vi "Dashboard Main.vi"() -> ()   [LabVIEW 2012]
uses:
  <vilib>/Rock Robotics/WPI/Camera/WPI_CameraWhite Balance Values.ctl
  <vilib>/event_ctls.llb/eventvkey.ctl
  <vilib>/Utility/config.llb/Read Key (String).vi
  <vilib>/Utility/config.llb/Read Key (I32).vi
  <vilib>/Utility/config.llb/Write Key (String).vi
  <vilib>/Utility/config.llb/Write Key (I32).vi
  <vilib>/Utility/inputDevices.llb/keyboardAcquire.vi
  Keys Pressed Global.vi
  <vilib>/Utility/inputDevices.llb/joystickAcquire.vi
  <vilib>/Utility/config.llb/NI_LVConfig.lvlib
panel:
  in  "Range":cluster{"Lower value":sgl, "Upper value":sgl}={"Lower value"=150.0, "Upper value"=255.0} {"Lower value" scale=0.0..255.0; "Upper value" scale=0.0..255.0}
  in  "Color Plane":i32(ring)=7 items=["Red", "Green", "Blue", "Hue", "Saturation", "Luminance", "Value", "Intensity"]
  out "Battery Value":dbl(slide) scale=0.0..14.0 scale format="%#_2e"
  out "Battery":sgl(graph)
  in  "Camera Settings":T1={"Frate Rate"=30, "Compression"=30, "Size"=0} {"Frate Rate" scale=1.0..30.0; "Size" items=["640x480", "320x240", "160x120"]}
  out "Mode":T2(ring)=enum."Auto Disabled"
  out "Camera IP":string
  out "JS1 Z":dbl(slide) scale=-1.0..1.0 scale format="%#_2e"
  out "JS2 Z":dbl(slide) scale=-1.0..1.0 scale format="%#_2e"
  out "Joystick 1":cluster{"X":dbl, "Y":dbl}[](graph)
  out "Joystick 2":cluster{"X":dbl, "Y":dbl}[](graph)
  out "JS Buttons 1":T3
  out "JS Buttons 2":T3
  out "MotorSlide4":dbl(slide) scale=-1.0..1.0 scale format="%#_2e"
  out "MotorSlide3":dbl(slide) scale=-1.0..1.0 scale format="%#_2e"
  out "MotorSlide2":dbl(slide) scale=-1.0..1.0 scale format="%#_2e"
  in  "MotorName3":string="Front Left"
  in  "MotorName4":string="Front Right"
  in  "MotorName1":string="Rear Left"
  in  "MotorName2":string="Rear Right"
  out "MotorChart4":dbl(graph)
  out "MotorChart3":dbl(graph)
  out "MotorChart2":dbl(graph)
  out "MotorSlide1":dbl(slide) scale=-1.0..1.0 scale format="%#_2e"
  out "MotorChart1":dbl(graph)
  out "Robot IP":string
  in  "Dashboard Tab":T4(tab)
  in  "control feeder":bool
  in  "control flipper":bool
  in  "conveyer backward":bool
  in  "conveyer forward":bool
  in  "transfer backward":bool
  in  "transfer forward":bool
  in  "feeder":dbl(knob) scale=0.0..130.0
  in  "flipper":dbl(knob) scale=0.0..170.0
  in  "Checkbox 2":bool
  in  "Checkbox 1":bool
  in  "Slider 1":dbl(slide) scale=0.0..100.0
  out "keys pressed":T5(array[ring])
  out "Position of Target's Center (x, y)":dbl[](array[numeric])
  out "Distance to Targets Center [m]":dbl
  out "Processed Image":T6(plugin-control)
  out "Target Found":bool
  in  "Annotate":bool=TRUE
  in  "Slider":dbl(slide) scale=0.0..100.0 scale format="%#_3g"
  in  "On/Off":bool caption="Solenoid"
  in  "Test Name":u16(ring) items=["Select the test to run...", "Example Test", "-------------------------------", "List of tests is built in robot code.", "Replace with your own automated tests."]
  in  "Test Tree":string(tree)
  in  "Motor":cluster{"Value":dbl, "Enable":bool} {"Value" scale=-1.0..1.0 scale format="%#_3g"}
  out "Progress":T7 {"Test Progress" scale=0.0..100.0}
  in  "Rev/Fwd":cluster{"Forward":bool, "Reverse":bool}
  in  "Ring":u16(ring) items=["Auto", "Fixed indoor", "Fixed outdoor 1", "Fixed outdoor 2", "Fixed fluorescent 1", "Fixed fluorescent 2", "Hold current"]
  in  "Listbox":i32(listbox)
  out "Selected Target Info":T8
  in  "Target Choice":i8(knob) scale=0.0..2.0
  in  "Viewer":enum32{"Camera Image", "Map", "Variables"}(tab)
  in  "More Cam":bool
  out "Mbps":dbl format="%#.1g"
  in  "Enable":bool
  in  "DB Camera Config":bool
  out "Mbps":bool
  out "fps":dbl format="%#.1g"
  out "Image Error Message":string="Timeout in Camera Communications"
  out "Camera Image":T6(plugin-control)
  in  "1":bool
  in  "2":bool
  in  "3":bool
  in  "Pyramid":bool
  in  "Low":bool
  in  "Left":bool
  in  "Right":bool
  in  "High":bool
  out "Map":T6(plugin-control)
  out "Distance [Meter]":dbl
  out "Angle [Degrees]":dbl
  out "Latched Cordinates":i32[](array[numeric])
  out "Selected Goal":i32
  out "Selected Cordinates":i32[](array[numeric])
  out "Tree":string(tree)
  # "Drive & Motors"
  # "Robot IP:"
  # "feeder"
  # "transfer"
  # "flipper"
  # "conveyer belt"
  # "Customize by placing controls and indicators here and name to match\nDashboard Variables on robot."
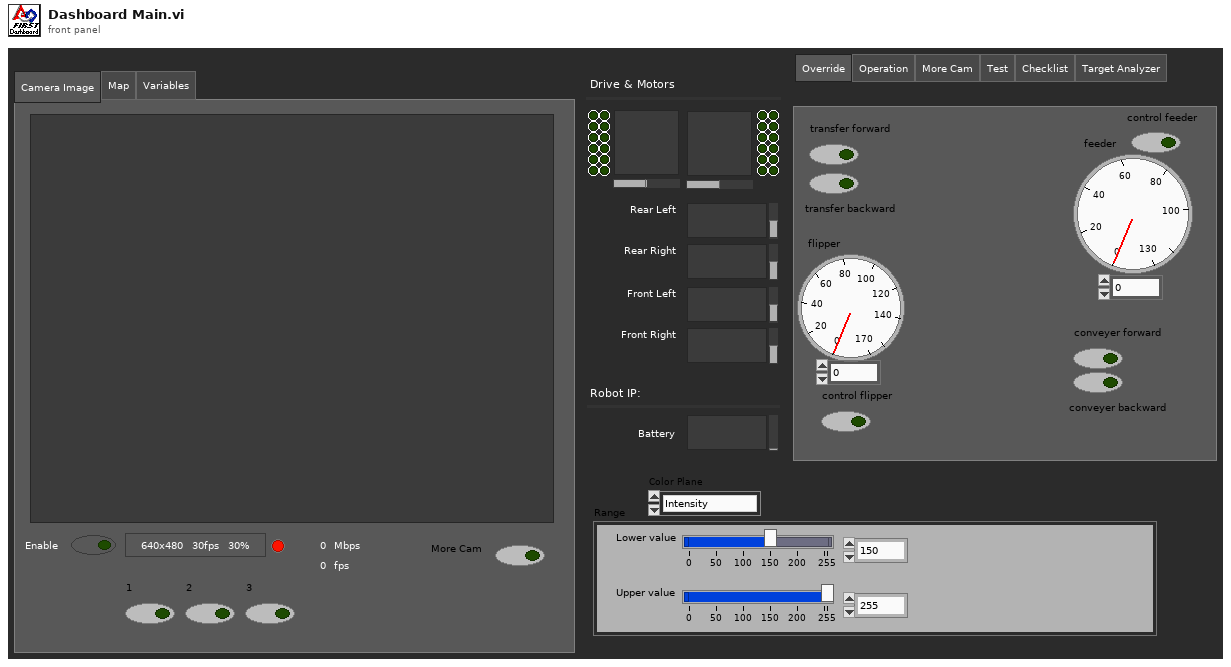
[diagram p1: front panel]
types:
  T1 = cluster{"Frate Rate":i32, "Compression":i32, "Size":u16}
  T2 = enum8{"Tele-Op Disabled", "Tele-Op Enabled", "Auto Disabled", "Auto Enabled", "Test Disabled", "Test Enabled", ""}
  T3 = cluster{bool, bool, bool, bool, bool, bool, bool, bool, bool, bool, bool, bool}
  T4 = enum32{"Override", "Operation", "More Cam", "Test", "Checklist", "Target Analyzer"}
  T5 = enum16{"0", "1", "2", "3", "4", "5", "6", "7", "8", "9", "A", "B", "C", "D", "E", "F", "G", "H", "I", "J", "K", "L", "M", "N", "O", "P", "Q", "R", "S", "T", "U", "V", "W", "X", "Y", "Z", "F1", "F2", "F3", "F4", "F5", "F6", "F7", "F8", "F9", "F10", "F11", "F12", "F13", "F14", "F15", "ADD", "BACK", "BACKSLASH", "CAPITAL", "COMMA", "DECIMAL", "DELETE", "DIVIDE", "DOWN", "END", "EQUALS", "ESCAPE", "GRAVE (`)", "HOME", "INSERT", "LBRACKET", "LCONTROL", "LEFT", "L ALT", "LSHIFT", "LWIN", "MINUS", "MULTIPLY", "NEXT", "NUMLOCK", "NUMPAD_0", "NUMPAD_1", "NUMPAD_2", "NUMPAD_3", "NUMPAD_4", "NUMPAD_5", "NUMPAD_6", "NUMPAD_7", "NUMPAD_8", "NUMPAD_9", "PAUSE", "PERIOD", "PRIOR (PG UP)", "RBRACKET", "RCONTROL", "RETURN", "RIGHT", "R ALT", "RSHIFT", "RWIN", "SCROLL", "SEMICOLON", "SLASH", "SPACE", "SUBTRACT", "TAB", "UP", "ENTER (num pad)", "' (quote)"}[]
  T6 = typedef "IMAQ Image.ctl" = refnum<image>
  T7 = cluster{"Test Progress":u8, "Test Progress Text":string}
  T8 = cluster{"Position":cluster{"X":dbl, "Y":dbl}, "Distance (m)":dbl, "Target Found?":bool}
  T9 = typedef "Image Type" = u32
  T10 = typedef "WPI_CameraWhite Balance Values.ctl" = enum16{"Auto", "Fixed indoor", "Fixed outdoor 1", "Fixed outdoor 2", "Fixed fluorescent 1", "Fixed fluorescent 2", "Hold current"}
  T11 = typedef "SkeletonTrackState.ctl" = enum32{"NotTracked", "PositionOnly", "Tracked"}
  T12 = cluster{"TrackingState":u8[], "Position":cluster{"x":sgl, "y":sgl, "z":sgl}, cluster{"x":sgl, "y":sgl, "z":sgl, sgl}[], "TrackState":T11}
  T13 = cluster{cluster{"ScaledToPercentRange":dbl, "ScaledToPercentRange":dbl, "ScaledToPercentRange":dbl}, cluster{bool, bool, bool}}[]
  T14 = cluster{cluster{"ScaledToPercentRange":dbl, "ScaledToPercentRange":dbl, "ScaledToPercentRange":dbl}, cluster{bool, bool, bool}}
  T15 = cluster{"ScaledToPercentRange":dbl, "ScaledToPercentRange":dbl, "ScaledToPercentRange":dbl}
  T16 = typedef "LVRectTypeDef.ctl" = cluster{"Left":i16, "Top":i16, "Right":i16, "Bottom":i16}
  T17 = cluster{"Competition mode":bool, "Robot Link":bool, "Autonomous":bool, "Enabled":bool, "E-Stop":bool, "Simulated":bool, "TestMode":bool, "Docked Window":bool}
  T18 = cluster{"Boolean Array[0]":bool, "Boolean Array[1]":bool, "Boolean Array[2]":bool, "Boolean Array[3]":bool, "Boolean Array[4]":bool, "Boolean Array[5]":bool, "Boolean Array[6]":bool, "Boolean Array[7]":bool, "Boolean Array[8]":bool, "Boolean Array[9]":bool, "Boolean Array[10]":bool, "Boolean Array[11]":bool}
  T19 = cluster{"Coordinates[0]":i32, "Coordinates[1]":i32, "Coordinates[2]":i32, "Coordinates[3]":i32, "Coordinates[4]":i32, "Coordinates[5]":i32, "Coordinates[6]":i32, "Coordinates[7]":i32, "Coordinates[8]":i32}
  T20 = cluster{"button 1":bool, "button 2":bool, "button 3":bool, "button 4":bool, "button 5":bool, "button 6":bool, "button 7":bool, "button 8":bool, "button 9":bool, "button 10":bool, "button 11":bool, "button 12":bool, "button 13":bool, "button 14":bool, "button 15":bool, "button 16":bool, "button 17":bool, "button 18":bool, "button 19":bool, "button 20":bool, "button 21":bool, "button 22":bool, "button 23":bool, "button 24":bool, "button 25":bool, "button 26":bool, "button 27":bool, "button 28":bool, "button 29":bool, "button 30":bool, "button 31":bool, "button 32":bool}
  T21 = enum16{"0", "1", "2", "3", "4", "5", "6", "7", "8", "9", "A", "B", "C", "D", "E", "F", "G", "H", "I", "J", "K", "L", "M", "N", "O", "P", "Q", "R", "S", "T", "U", "V", "W", "X", "Y", "Z", "F1", "F2", "F3", "F4", "F5", "F6", "F7", "F8", "F9", "F10", "F11", "F12", "F13", "F14", "F15", "ADD", "BACK", "BACKSLASH", "CAPITAL", "COMMA", "DECIMAL", "DELETE", "DIVIDE", "DOWN", "END", "EQUALS", "ESCAPE", "GRAVE (`)", "HOME", "INSERT", "LBRACKET", "LCONTROL", "LEFT", "L ALT", "LSHIFT", "LWIN", "MINUS", "MULTIPLY", "NEXT", "NUMLOCK", "NUMPAD_0", "NUMPAD_1", "NUMPAD_2", "NUMPAD_3", "NUMPAD_4", "NUMPAD_5", "NUMPAD_6", "NUMPAD_7", "NUMPAD_8", "NUMPAD_9", "PAUSE", "PERIOD", "PRIOR (PG UP)", "RBRACKET", "RCONTROL", "RETURN", "RIGHT", "R ALT", "RSHIFT", "RWIN", "SCROLL", "SEMICOLON", "SLASH", "SPACE", "SUBTRACT", "TAB", "UP", "ENTER (num pad)", "' (quote)"}
  T22 = enum32{"Override", "Operation", "More Cam", "Test", "Checklist"}
  T23 = typedef "WPI_CameraDevRef.ctl" = cluster{"Camera Address":string, "CameraStatus":errorcluster, "Acquire Image Notifier":refnum<notifier>}
  T24 = typedef "NI_LVConfig.lvlib/Config Data RefNum.ctl" = refnum<k1>
  T25 = cluster{"Center Position":cluster{"X":dbl, "Y":dbl}, "Distance (ft)":dbl, "Center":bool}[]
  T26 = cluster{cluster{"Left":dbl, "Top":dbl, "Right":dbl, "Bottom":dbl}, "Scores":dbl[], cluster{"Long":dbl, "Short":dbl}}
  T27 = typedef "eventvkey.ctl" = enum16{"ASCII", "Enter", "Return", "Shift", "Ctrl", "Alt", "Cmd", "Opt", "Caps", "NumLock", "Clear", "Break", "Up", "Down", "Left", "Right", "Insert", "Delete", "Home", "End", "PageUp", "PageDown", "Escape", "Help", "Pause", "ScrollLock", "F1", "F2", "F3", "F4", "F5", "F6", "F7", "F8", "F9", "F10", "F11", "F12", "F13", "F14", "F15", "F16", "F17", "F18", "F19", "F20", "F21", "F22", "F23", "F24", "Play", "VolumeUp", "VolumeDown", "Mute", "Two Byte Char"}
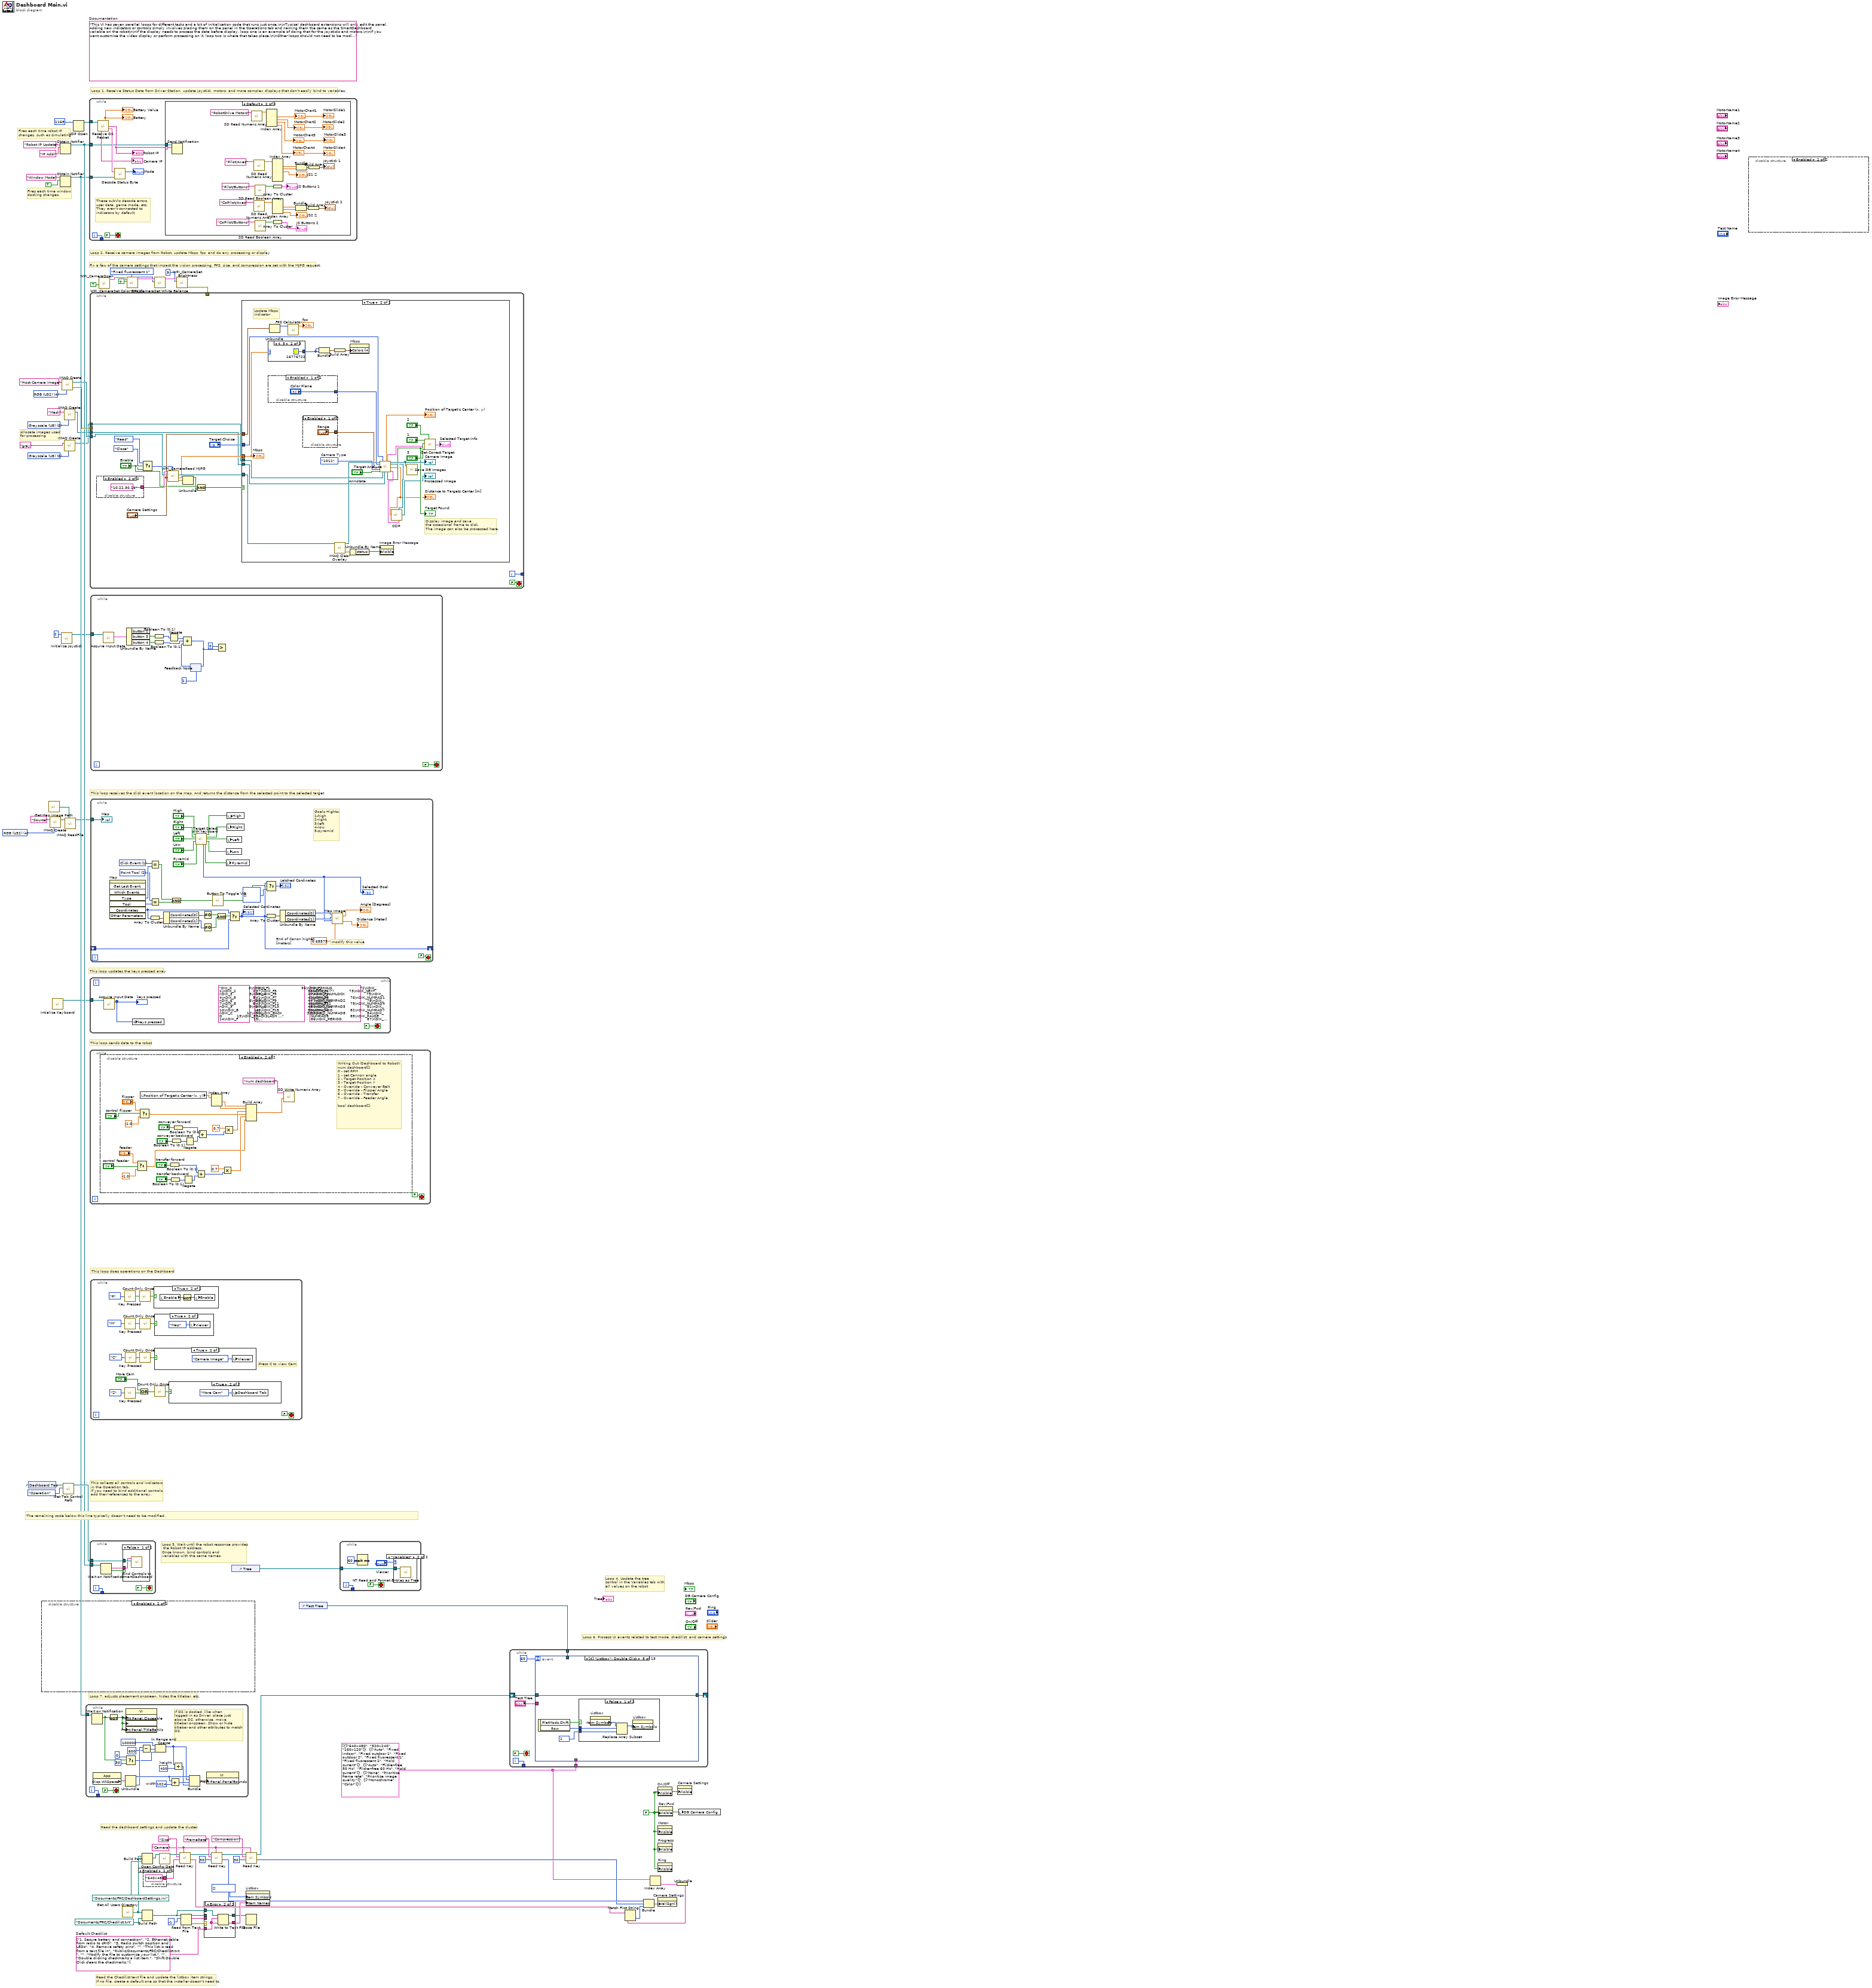
[diagram p0: block diagram]
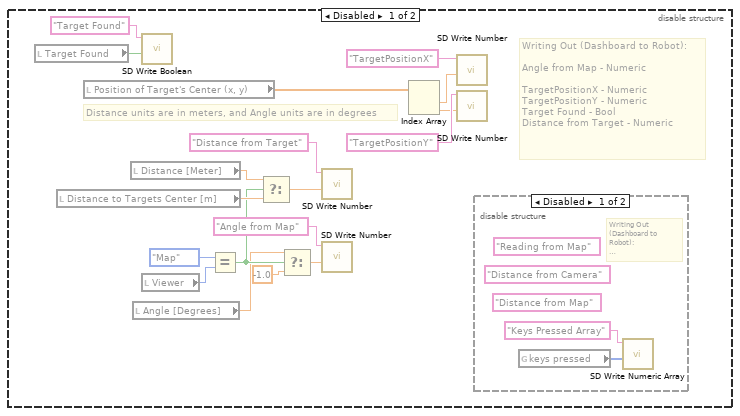
[diagram p6: hidden frame]
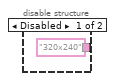
[diagram p8: hidden frame]
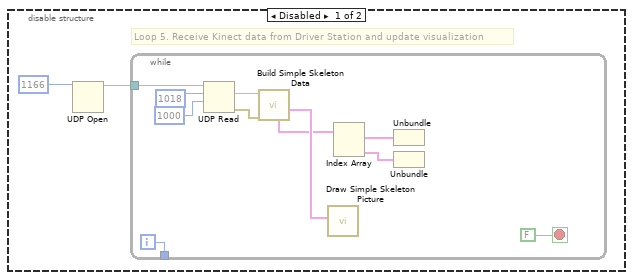
[diagram p9: hidden frame]
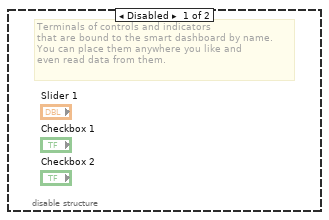
[diagram p10: hidden frame]
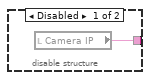
[diagram p12: hidden frame]
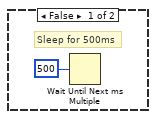
[diagram p13: hidden frame]
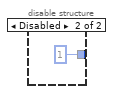
[diagram p14: hidden frame]
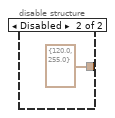
[diagram p15: hidden frame]
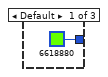
[diagram p16: hidden frame]
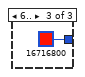
[diagram p17: hidden frame]
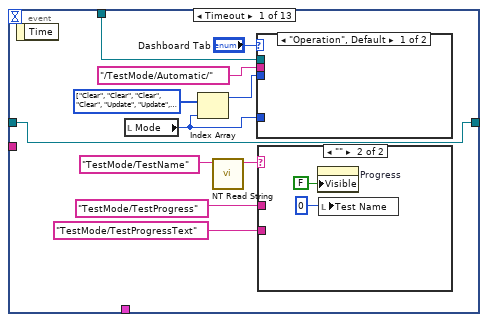
[diagram p19: hidden frame]
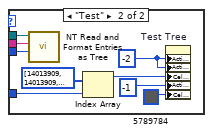
[diagram p20: hidden frame]
diagram:
  w5 = T9 0 items=["Grayscale (U8)", "Grayscale (I16)", "Grayscale (SGL)", "Complex (CSG)", "RGB (U32)", "HSL (U32)", "RGB (U64)", "Grayscale (U16)"] ("Image Type")
  w8 = T9 0 items=["Grayscale (U8)", "Grayscale (I16)", "Grayscale (SGL)", "Complex (CSG)", "RGB (U32)", "HSL (U32)", "RGB (U64)", "Grayscale (U16)"] ("Image Type")
  w14 = T9 4 items=["Grayscale (U8)", "Grayscale (I16)", "Grayscale (SGL)", "Complex (CSG)", "RGB (U32)", "HSL (U32)", "RGB (U64)", "Grayscale (U16)"] ("Image Type")
  w43 = "Camera"
  w35 = cluster{string[]}[] [{["640x480", "320x240", "160x120"]}, {["Auto", "Fixed indoor", "Fixed outdoor 1", "Fixed outdoor 2", "Fixed fluorescent 1", "Fixed fluorescent 2", "Hold current"]}, {["Auto", "Flicker-free 50 Hz", "Flicker-free 60 Hz", "Hold current"]}, {["None", "Prioritize frame rate", "Prioritize image quality"]}, {["Monochrome", "Color"]}]
  w51 = string[] ["1. Secure battery and connection", "2. Ethernet cable from radio to cRIO", "3. Radio switch position and LEDs", "4. Remove safety pins", "", "This list is read from a text file in", "Public/Documents/FRC/Checklist.txt.", "", "Modify the file to customize your list.", "", "Double clicking checkmarks a list item.", "Shift Double Click clears the checkmarks."]  # Default Checklist
  w49 = FALSE ("Visible")
  (unwired) "This VI has seven parallel loops for different tasks and a bit of initialization code that runs just once.\n\nTypical dashboard extensions will only edit the panel. Adding new indicators or controls simply involves placing them on the panel in the Operations tab and naming them the same as the SmartDashboard variable on the robot\n\nIf the display needs to process the data before display, loop one is an example of doing that for the joysticks and motors.\n\nIf you want customize the video display or perform processing on it, loop two is where that takes place.\n\nOther loops should not need to be modified. They are pretty standard, and document the task they perform."  # Documentation
  w70 = T9 4 items=["Grayscale (U8)", "Grayscale (I16)", "Grayscale (SGL)", "Complex (CSG)", "RGB (U32)", "HSL (U32)", "RGB (U64)"] ("Image Type")
  # "Allocate images used\nfor processing"
  # "This loop does operations on the Dashboard"
  # "This loop sends data to the robot"
  # "This loop updates the keys pressed array"
  # "This loop receives the click event location on the map. And returns the distance from the selected point to the selected target"
  # "Fix a few of the camera settings that impact the vision processing. FPS, size, and compression are set with the MJPG request."
  # "Fires each time robot IP\nchanges, such as simulating"
  # "Fires each time window\ndocking changes."
  # "Read the Checklist text file and update the listbox item strings.\nIf no file, create a default one so that the installer doesn't need to."
  # "This collects all controls and indicators\nin the Operation tab.\nIf you need to bind additional controls,\nadd their references to the array."
  # "The remaining code below this line typically doesn't need to be modified."
  # "Loop 6. Process UI events related to test mode, checklist, and camera settings"
  # "Read the dashboard settings and update the cluster."
  # "Loop 4. Update the tree\ncontrol in the Variables tab with\nall values on the robot"
  # "Loop 3. Wait until the robot response provides\n the Robot IP address.\nOnce known, bind controls and\nvariables with the same names."
  # "Loop 7. adjusts placement onscreen, hides the titlebar, etc."
  # "Loop 1. Receive Status Data from Driver Station, update joystick, motors, and more complex displays that don't easily bind to variables."
  # "Loop 2. Receive camera images from Robot, update Mbps, fps, and do any processing or display"
  n1 = control-ref of="Dashboard Tab"() -> (w65:refnum<vi>)
  n2 = disable-structure shown="Enabled" {
    frame Disabled {
      # "Loop 5. Receive Kinect data from Driver Station and update visualization"
      n3 = UDP Open(11:u16 1166 ("port")) -> (port=w73:refnum<k16>)  [unwired: 2 in, 4 out]
      n4 = while {
        tunnel: w73 -> [w89]
        tunnel: [w76] -> _
        i -> [w76]
        stop <- FALSE stop-if-true
        n5 = UDP Read(connection ID=w89, max size (548)=1018 ("bytes to read"), timeout ms (25000)=1000) -> (data out=w84:string, error out=w75:errorcluster)  [unwired: 1 in, 3 out]
        n6 = call "Build Simple Skeleton Data.vi"("error in (no error)"=w75, "data in"=w84) -> ("Skeleton Data"=w85:T12, "NumPlayers"=w87:i8, "Version String"=w88:string, "Simple Joystick Info"=w82:T13)  [unwired: 5 in, 1 out]
        n7 = call "Draw Simple Skeleton Picture.vi"("Simple Skeleton"=w85) -> ("new picture out"=w86:picture)  [unwired: 10 in]
        n8 = Index Array(array=w82) -> (element #1=w81:T14, element #2=w80:T14)  [unwired: 2 in]
        n9 = Unbundle(w81) -> (w79:T15)  [unwired: 1 out]
        n10 = Unbundle(w80) -> (w78:T15, w77:cluster{bool, bool, bool})
      }
    }
    frame Enabled {
    }
  }
  n11 = call "Get Map Image Path.vi"() -> ("Image Path"=w10:path)  [unwired: 1 in]
  n12 = call "IMAQ Create"("Image Name"="Source", "Image Type"=w14) -> ("New Image"=w12:T6)  [unwired: 2 in, 2 out]
  n13 = call <vilib>:"Intialize Keyboard.vi"() -> ("device ID"=w9:refnum<k1>)  [unwired: 10 in, 1 out]
  n14 = Obtain Notifier(name (unnamed)="Robot IP Update", notification data type="IP Addr" ("name (unnamed)")) -> (notifier out=w62:refnum<notifier>)  [unwired: 2 in, 2 out]
  n15 = Obtain Notifier(name (unnamed)="Window Mode", notification data type=TRUE) -> (notifier out=w55:refnum<notifier>)  [unwired: 2 in, 2 out]
  n16 = call <vilib>:"Initialize Joystick.vi"("device index"=2) -> ("device ID"=w2:refnum<k1>)  [unwired: 9 in, 1 out]
  n17 = call "IMAQ Create"("Image Name"="Host Camera Image", "Image Type"=w70) -> ("New Image"=w68:T6, "error out"=w67:errorcluster)  [unwired: 2 in, 1 out]
  n18 = call <vilib>:"Get Tab Control Refs.vi"("Page Index"=enum32{"Operation", "Test"}."Operation" ("Dashboard Tab"), "TabControl in"=w65) -> ("ControlsOnPage"=w66:refnum<vi>[])  [unwired: 9 in]
  n19 = call "IMAQ Create"("Image Name"="Mask", "Image Type"=w5) -> ("New Image"=w4:T6)  [unwired: 2 in, 2 out]
  n20 = call "IMAQ Create"("Image Name"="gray", "Image Type"=w8) -> ("New Image"=w3:T6)  [unwired: 2 in, 2 out]
  n21 = call "IMAQ ReadFile"("File Path"=w10, "Image"=w12) -> ("Image Out"=w13:T6)  [unwired: 5 in, 4 out]
  n22 = UDP Open(11:u16 1165 ("port")) -> (port=w71:refnum<k16>)  [unwired: 2 in, 4 out]
  n23 = while {
    tunnel: w55 -> [w110]
    tunnel: [w108] -> _
    i -> [w108]
    stop <- FALSE stop-if-true
    w100 = 1024  # width
    w103 = 400  # height
    # "If DS is docked, like when\nlogged in as Driver, place just\nabove DS, otherwise, move\ntitlebar onscreen. Show or hide\ntitlebar and other attributes to match\nDS."
    n24 = Wait on Notification(notifier=w110) -> (notification=w95:bool)  [unwired: 3 in, 3 out]
    n25 = property class="App"() -> ("Disp.WkSpace"=w106:T16)  [unwired: 2 in, 2 out]
    n26 = Not(x=w95) -> (.not. x?=w109:bool)
    n27 = Unbundle(w106) -> ("Left"=w104:i16, "Bottom"=w101:i16)  [unwired: 2 out]
    n28 = Select(t=0, s=w95, f=30) -> (s? t:f=w94:i32)
    n29 = property class="VI"("Front Panel.Closeable"=w109, "Front Panel.Minimizeable"=w109, "Front Panel.TitleBarVis"=w109) -> ()  [unwired: 2 in, 2 out]
    n30 = Subtract(x=w101, y=600) -> (x-y=w98:i32)
    n31 = In Range and Coerce(upper limit=100000, x=w98, lower limit=w94) -> (coerced(x)=w92:i32)  [unwired: 1 out]
    n32 = Add(x=w104, y=w100) -> (x+y=w105:i32)
    n33 = Add(x=w92, y=w103) -> (x+y=w102:i32)
    n34 = Bundle("Left"=w104, w92, w105, w102) -> (w107:cluster{"Left":i16, i32, i32, i32})  [unwired: 1 out]
    n35 = property class="VI"("Front Panel.PanelBounds"=w107) -> ()  [unwired: 2 in, 2 out]
  }
  n36 = while {
    tunnel: w71 -> [w119]
    tunnel: w62 -> [w113]
    tunnel: w55 -> [w117]
    tunnel: [w114] -> _
    i -> [w114]
    stop <- FALSE stop-if-true
    # "These subVIs decode errors, user data, game mode, etc.\nThey aren't connected to indicators by default"
    n37 = call "Receive DS Packet.vi"("Recv Socket"=w119) -> ("Battery"=→"Battery" →"Battery Value":sgl, "Robot IP Address"=w112:string, "Status"=w120:T17, "Camera IP Address"=→"Camera IP":string)  [unwired: 1 in, 10 out]
    "Robot IP" <- w112
    n38 = call "Decode Status Byte.vi"("Window Mode Notifier"=w117, "Status"=w120) -> ("Mode"=→"Mode":T2)  [unwired: 1 out]
    n39 = case shown="Default" w112 {
      selector: w112 -> [_ w122]
      tunnel: w113 -> [_ w123]
      frame "0.0.0.0" {
        # "Robot not responding, don't poll the variables"
      }
      frame Default {
        n40 = Send Notification(notification=w122, notifier=w123) -> ()  [unwired: 1 in, 2 out]
        n41 = call <vilib>:"SD Read Numeric Array.vi"("Name"="RobotDrive Motors") -> ("Numeric Array"=w146:dbl[])  [unwired: 8 in, 2 out]
        n42 = call <vilib>:"SD Read Numeric Array.vi"("Name"="Pilot/Axes") -> ("Numeric Array"=w139:dbl[])  [unwired: 8 in, 2 out]
        n43 = call <vilib>:"SD Read Numeric Array.vi"("Name"="CoPilot/Axes") -> ("Numeric Array"=w133:dbl[])  [unwired: 8 in, 2 out]
        n44 = call <vilib>:"SD Read Boolean Array.vi"("Name"="Pilot/Buttons") -> ("Boolean Array"=w141:bool[])  [unwired: 8 in, 2 out]
        n45 = call <vilib>:"SD Read Boolean Array.vi"("Name"="CoPilot/Buttons") -> ("Boolean Array"=w132:bool[])  [unwired: 8 in, 2 out]
        n46 = Index Array(array=w146) -> (element #1=→"MotorChart1" →"MotorSlide1":dbl, element #2=→"MotorSlide2" →"MotorChart2":dbl, element #3=→"MotorChart3" →"MotorSlide3":dbl, element #4=→"MotorChart4" →"MotorSlide4":dbl)  [unwired: 4 in]
        n47 = Array To Cluster(array=w141) -> (cluster=→"JS Buttons 1":T18)
        n48 = Array To Cluster(array=w132) -> (cluster=→"JS Buttons 2":T18)
        n49 = Index Array(array=w139) -> (element #1=w136:dbl, element #2=w137:dbl, element #3=→"JS1 Z":dbl)  [unwired: 6 in, 3 out]
        n50 = Index Array(array=w133) -> (element #1=w128:dbl, element #2=w127:dbl, element #3=→"JS2 Z":dbl)  [unwired: 3 in]
        n51 = Bundle("Numeric"=w128, "Numeric"=w127) -> (w129:cluster{"Numeric":dbl, "Numeric":dbl})  [unwired: 1 in]
        n52 = Bundle("Numeric"=w136, "Numeric"=w137) -> (w135:cluster{"Numeric":dbl, "Numeric":dbl})  [unwired: 1 in]
        n53 = Build Array(w129) -> (→"Joystick 2":cluster{"Numeric":dbl, "Numeric":dbl}[])
        n54 = Build Array(w135) -> (→"Joystick 1":cluster{"Numeric":dbl, "Numeric":dbl}[])
      }
    }
  }
  n55 = while {
    stop <- FALSE stop-if-true
    n56 = disable-structure shown="Enabled" {
      frame Disabled {
        # "Writing Out (Dashboard to Robot):\n\nAngle from Map - Numeric\n\nTargetPositionX - Numeric\nTargetPositionY - Numeric\nTarget Found - Bool\nDistance from Target - Numeric"
        # "Distance units are in meters, and Angle units are in degrees"
        n57 = local read "Target Found"() -> (w159:bool)
        n58 = local read "Distance to Targets Center [m]"() -> (w156:dbl)
        n59 = local read "Position of Target's Center (x, y)"() -> (w162:dbl[])
        n60 = local read "Distance [Meter]"() -> (w157:dbl)
        n61 = local read "Angle [Degrees]"() -> (w153:dbl)
        n62 = call <vilib>:"SD Write Boolean.vi"("Boolean"=w159, "Name"="Target Found") -> ()  [unwired: 8 in, 2 out]
        n63 = local read "Viewer"() -> (w166:enum32{"Camera Image", "Map", "Variables"})
        n64 = Equal?(x=enum32{"Camera Image", "Map", "Variables"}."Map" ("Viewer"), y=w166) -> (x = y?=w154:bool)
        n65 = Select(t=w157, s=w154, f=w156) -> (s? t:f=w155:dbl)
        n66 = Select(t=w153, s=w154, f=-1.0) -> (s? t:f=w152:dbl)
        n67 = call <vilib>:"SD Write Number.vi"("Numeric"=w155, "Name"="Distance from Target") -> ()  [unwired: 8 in, 2 out]
        n68 = call <vilib>:"SD Write Number.vi"("Numeric"=w152, "Name"="Angle from Map") -> ()  [unwired: 8 in, 2 out]
        n69 = Index Array(array=w162) -> (element #1=w161:dbl, element #2=w160:dbl)  [unwired: 2 in]
        n70 = call <vilib>:"SD Write Number.vi"("Numeric"=w161, "Name"="TargetPositionX") -> ()  [unwired: 8 in, 2 out]
        n71 = call <vilib>:"SD Write Number.vi"("Numeric"=w160, "Name"="TargetPositionY") -> ()  [unwired: 8 in, 2 out]
        n72 = disable-structure shown="Disabled" {
          frame Disabled {
            (unwired) "Reading from Map" ("Name")
            (unwired) "Distance from Camera" ("Name")
            (unwired) "Distance from Map" ("Name")
            # "Writing Out (Dashboard to Robot):\n\nKeys Pressed Array - Numeric Array\n\nReading from Map - Bool\nDistance from Map - Numeric\nAngle from Map - Numeric\n\nTargetPositionX - Numeric\nTargetPositionY - Numeric\nCenter Target - Bool\nDistance from Camera - Numeric"
            n73 = global read "Keys Pressed Global.vi" "keys pressed"() -> (w169:T5)
            n74 = call <vilib>:"SD Write Numeric Array.vi"("Numeric Array"=w169, "Name"="Keys Pressed Array") -> ()  [unwired: 8 in, 2 out]
          }
          frame Enabled {
          }
        }
      }
      frame Enabled {
        # "Writing Out (Dashboard to Robot):\nnum dashboard[]:\n0 - set RPM\n1 - set Cannon angle\n2 - Target Position X\n3 - Target Position Y\n4 - Override - Conveyer Belt\n5 - Override - Flipper Angle \n6 - Override - Transfer\n7 - Override - Feeder Angle\n\nbool dashboard[]:"
        n75 = Select(t="feeder", s="control feeder", f=-1.0) -> (s? t:f=w172:dbl)
        n76 = Select(t="flipper", s="control flipper", f=-1.0) -> (s? t:f=w177:dbl)
        n77 = local read "Position of Target's Center (x, y)"() -> (w198:dbl[])
        n78 = Boolean To (0,1)(Boolean="transfer forward") -> (0, 1=w187:i16)
        n79 = Boolean To (0,1)(Boolean="transfer backward") -> (0, 1=w189:i16)
        n80 = Boolean To (0,1)(Boolean="conveyer backward") -> (0, 1=w190:i16)
        n81 = Boolean To (0,1)(Boolean="conveyer forward") -> (0, 1=w185:i16)
        n82 = Negate(x=w189) -> (-x=w188:i16)
        n83 = Negate(x=w190) -> (-x=w186:i16)
        n84 = Add(x=w187, y=w188) -> (x+y=w181:i16)
        n85 = Add(x=w185, y=w186) -> (x+y=w183:i16)
        n86 = Index Array(array=w198) -> (element #1=w197:dbl, element #2=w196:dbl)  [unwired: 2 in]
        n87 = Multiply(x=0.7, y=w181) -> (x*y=w179:dbl)
        n88 = Multiply(x=0.7, y=w183) -> (x*y=w180:dbl)
        n89 = Build Array(w197, w196, w180, w177, w179, w172) -> (w195:dbl[])
        n90 = call <vilib>:"SD Write Numeric Array.vi"("Numeric Array"=w195, "Name"="num dashboard") -> ()  [unwired: 8 in, 2 out]
      }
    }
  }
  n91 = while {
    tunnel: w9 -> [w202]
    stop <- FALSE stop-if-true
    (unwired) "DIK_MINUS                       72\nDIK_MULTIPLY (*)             73\nDIK_NEXT                          74\nDIK_NUMLOCK                  75\nDIK_NUMPAD0                  76\nDIK_NUMPAD1                  77\nDIK_NUMPAD2                  78\nDIK_NUMPAD3                  79\nDIK_NUMPAD4                  80\nDIK_NUMPAD5                  81\nDIK_NUMPAD6                  82\nDIK_NUMPAD7                  83\nDIK_NUMPAD8                  84\nDIK_NUMPAD9                  85\nDIK_PAUSE                       86\nDIK_PERIOD                     87\nDIK_PRIOR (pg up)           88\nDIK_RBRACKET ( ] )          89\nDIK_RCONTROL               90\nDIK_RETURN                    91\nDIK_RIGHT                       92\nDIK_RMENU (R ALT)         93\nDIK_RSHIFT (R shift)       94\nDIK_RWIN (R win)            95\nDIK_SCROLL                     96\nDIK_SEMICOLON              97\nDIK_SLASH                       98\nDIK_SPACE                       99\nDIK_SUBTRACT               100\nDIK_TAB                          101\nDIK_UP                            102\nDIR_ENTER(NUM)           103\nDIR_APOSTROPHY         104"
    (unwired) "DIK_F1                          36\nDIK_F2                          37\nDIK_F3                          38\nDIK_F4                          39\nDIK_F5                          40\nDIK_F6                          41\nDIK_F7                          42\nDIK_F8                          43\nDIK_F9                          44 \nDIK_F10                        45\nDIK_F11                        46\nDIK_F12                        47\nDIK_F13                        48 \nDIK_F14                        49\nDIK_F15                        50\nDIK_ADD                       51\nDIK_BACK                     52\nDIK_BACKSLASH           53\nDIK_CAPITAL                54\nDIK_COMMA                 55\nDIK_DECIMAL               56\nDIK_DELETE                  57\nDIK_DIVIDE                  58\nDIK_DOWN                   59\nDIK_END                       60\nDIK_EQUALS                 61\nDIK_ESCAPE                 62\nDIK_GRAVE (`)             63\nDIK_HOME                    64\nDIK_INSERT                  65\nDIK_LBRACKET             66\nDIK_LCONTROL            67\nDIK_LEFT                      68\nDIK_LMENU (L ALT)      69\nDIK_LSHIFT                  70\nDIK_LWIN                    71\n\n\n\n\n\n\n"
    (unwired) "DIK_0              0\nDIK_1              1\nDIK_2              2\nDIK_3              3\nDIK_4              4\nDIK_5              5\nDIK_6              6\nDIK_7              7\nDIK_8              8\nDIK_9              9\nDIK_A            10\nDIK_B             11\nDIK_C            12\nDIK_D            13\nDIK_E             14\nDIK_F             15\nDIK_G            16\nDIK_H            17\nDIK_I             18\nDIK_J             19\nDIK_K             20\nDIK_L             21\nDIK_M            22\nDIK_N            23\nDIK_O            24\nDIK_P             25\nDIK_Q            26\nDIK_R            27\nDIK_S             28\nDIK_T             29\nDIK_U            30\nDIK_V             31\nDIK_W           32\nDIK_X             33\nDIK_Y             34\nDIK_Z             35\n\n"
    n92 = call-poly <vilib>:"Acquire Input Data.vi"("device ID"=w202) -> ("keys pressed"=w200:T5)  [unwired: 2 in, 16 out]
    "keys pressed" <- w200
    n93 = global write "Keys Pressed Global.vi" "keys pressed"(w200) -> ()
  }
  n94 = while {
    tunnel: w66 -> [w208]
    tunnel: w62 -> [w205]
    tunnel: [w203] -> _
    i -> [w203]
    stop <- FALSE stop-if-true
    n95 = Wait on Notification(notifier=w205) -> (notification=w204:string, timed out?=w206:bool)  [unwired: 3 in, 2 out]
    n96 = case shown="False" w206 {
      tunnel: w208 -> [w210 _]
      tunnel: w204 -> [w209 _]
      frame False {
        n97 = call <vilib>:"Bind Controls to SmartDashboard.vi"("Bound Control Refs"=w210, "Server IP Address"=w209) -> ()  [unwired: 10 in]
      }
      frame True {
      }
    }
  }
  n98 = while {
    tunnel: w13 -> [w242]
    shift-right: [w229] -> _
    shift-left: _ -> [w233]
    stop <- FALSE stop-if-true
    w226 = 0.68575  # End of Canon highet [meters]
    w243 = 2 items=["None", "Selection Tool", "Point Tool", "Line Tool", "Rectangle Tool", "Oval Tool", "Polygon Tool", "ClosedFreehandTool", "Annulus Tool", "Rotated Rectangle Tool", "Zoom Tool", "Pan Tool", "Polyline Tool", "Freehand Tool"] ("Tool")
    w244 = 1 items=["No Event"=0, "Click Event"=1, "Draw Event"=2, "Size Event"=4, "Scroll Event"=5, "Double Click Event"=8] ("Type")
    # "Goals Hights:\n1-high\n2-right\n3-left\n4-low\n5-pyramid"
    # "modify this value"
    n99 = invoke on="Map" class="ImageControl" method="Get Last Event"() -> ("Type"=w245:i32, "Tool"=w248:i32, "Coordinates"=w234:i32[])  [unwired: 8 in, 5 out]
    n100 = Equal?(x=w244, y=w245) -> (x = y?=w246:bool)
    n101 = Equal?(x=w243, y=w248) -> (x = y?=w247:bool)
    n102 = Array To Cluster(array=w234) -> (cluster=w240:T19)
    n103 = Unbundle By Name(w240) -> ("Coordinates[0]"=w238:i32, "Coordinates[1]"=w236:i32)
    n104 = And(x=w246, y=w247) -> (x .and. y?=w218:bool)
    n105 = call "Target Select with keyboard.vi"("High"="High", "Right"="Right", "Left"="Left", "Low"="Low", "Pyramid"="Pyramid") -> ("1"=w211:bool, "2"=w212:bool, "3"=w213:bool, "4"=w214:bool, "Selected Goal"=w216:i32, "5"=w215:bool)  [unwired: 5 in]
    "Selected Goal" <- w216
    n106 = Not Equal To 0?(x=w238) -> (x != 0?=w239:bool)
    n107 = Not Equal To 0?(x=w236) -> (x != 0?=w237:bool)
    n108 = call "Button To Toggle Vr3.vi"("InValue"=w218) -> ("Result"=w217:bool)
    n109 = And(x=w239, y=w237) -> (x .and. y?=w235:bool)
    n110 = local write "Pyramid"(w215) -> ()
    n111 = local write "Low"(w214) -> ()
    n112 = local write "Right"(w212) -> ()
    n113 = local write "Left"(w213) -> ()
    n114 = local write "High"(w211) -> ()
    n115 = Select(t=w234, s=w235, f=w233) -> (s? t:f=w229:i32[])
    "Selected Cordinates" <- w229
    n116 = Array To Cluster(array=w229) -> (cluster=w230:T19)
    n117 = Select(t=w229, s=w217, f=i32[] [] ("Coordinates")) -> (s? t:f=→"Latched Cordinates":i32[])
    n118 = Unbundle By Name(w230) -> ("Coordinates[0]"=w227:i32, "Coordinates[1]"=w228:i32)
    n119 = call "Map Image.vi"("End of Canon highet [meters]"=w226, "Goal Number"=w216, "Y[Pixels]"=w228, "X [Pixels]"=w227) -> ("Distance [Meter]"=→"Distance [Meter]":dbl, "Angel [Degrees]"=→"Angle [Degrees]":dbl)
    "Map" <- w242
  }
  n120 = while {
    tunnel: w2 -> [w259]
    stop <- FALSE stop-if-true
    n121 = call-poly <vilib>:"Acquire Input Data.vi"("device ID"=w259) -> ("button info"=w258:T20)  [unwired: 2 in, 16 out]
    n122 = Unbundle By Name(w258) -> ("button 3"=w257:bool, "button 4"=w256:bool)  [unwired: 1 out]
    n123 = Boolean To (0,1)(Boolean=w257) -> (0, 1=w255:i16)
    n124 = Boolean To (0,1)(Boolean=w256) -> (0, 1=w253:i16)
    n125 = Negate(x=w255) -> (-x=w254:i16)
    n126 = feedback #1(i16 1) -> (w251:i16)
    n127 = Compound Arithmetic op=ADD(w254, w253, w251) -> (w250:i16)
    n128 = feedback-in #1(w250) -> ()
    n129 = Greater?(x=i16 0, y=w250) -> ()  [unwired: 1 out]
  }
  n130 = while {
    stop <- FALSE stop-if-true
    # "Press C to view Cam"
    n131 = call "Key Pressed.vi"("key to be pressed"=T21."P") -> ("Was this key pressed"=w262:bool)
    n132 = call "Key Pressed.vi"("key to be pressed"=T21."M") -> ("Was this key pressed"=w265:bool)
    n133 = call "Key Pressed.vi"("key to be pressed"=T21."Z") -> ("Was this key pressed"=w267:bool)
    n134 = call "Key Pressed.vi"("key to be pressed"=T21."C") -> ("Was this key pressed"=w272:bool)
    n135 = Or(x="More Cam", y=w267) -> (x .or. y?=w269:bool)
    n136 = call "Count Only Once.vi"("InValue"=w262) -> ("Result"=w261:bool)
    n137 = call "Count Only Once.vi"("InValue"=w265) -> ("Result"=w266:bool)
    n138 = call "Count Only Once.vi"("InValue"=w272) -> ("Result"=w271:bool)
    n139 = case shown="True" w261 {
      frame False {
      }
      frame True {
        n140 = local read "Enable"() -> (w276:bool)
        n141 = Not(x=w276) -> (.not. x?=w277:bool)
        n142 = local write "Enable"(w277) -> ()
      }
    }
    n143 = case shown="True" w266 {
      frame False {
      }
      frame True {
        n144 = local write "Viewer"(enum32{"Camera Image", "Map", "Variables"}."Map" ("t")) -> ()
      }
    }
    n145 = case shown="True" w271 {
      frame False {
      }
      frame True {
        n146 = local write "Viewer"(enum32{"Camera Image", "Map", "Variables"}."Camera Image" ("t")) -> ()
      }
    }
    n147 = call "Count Only Once.vi"("InValue"=w269) -> ("Result"=w273:bool)
    n148 = case shown="True" w273 {
      frame False {
      }
      frame True {
        n149 = local write "Dashboard Tab"(T22."More Cam" ("Dashboard Tab")) -> ()
      }
    }
  }
  n150 = call <vilib>:"WPI_CameraOpen.vi"("Disallow Simulation"=TRUE) -> ("CameraDevRef"=w22:T23)  [unwired: 9 in, 1 out]
  n151 = call "Get All Users Directory.vi"() -> ("All User Path"=w48:path)
  n152 = call <vilib>:"WPI_CameraSet Color Enable.vi"("Color Enabled"=TRUE, "CameraDevRef"=w22) -> ("CameraDevRef Out"=w20:T23)  [unwired: 8 in, 1 out]
  n153 = Build Path(base path=w48, name or relative path=path "Documents/FRC/DashboardSettings.ini") -> (appended path=w47:path)
  n154 = Build Path(base path=w48, name or relative path=path "Documents/FRC/Checklist.txt") -> (appended path=w52:path)
  n155 = disable-structure shown="Enabled" {
    disable-tunnel: ["320x240" "640x480"] -> w44
    frame Disabled {
    }
    frame Enabled {
    }
  }
  n156 = call <vilib>:"WPI_CameraSet White Balance.vi"("White Balance"=WPI_CameraWhite_Balance_Values."Fixed fluorescent 1", "CameraDevRef"=w20) -> ("CameraDevRef Out"=w18:T23)  [unwired: 8 in, 1 out]
  n157 = call <vilib>:"Open Config Data.vi"("configuration file path"=w47) -> ("refnum"=w46:T24)  [unwired: 8 in, 2 out]
  n158 = call <vilib>:"WPI_CameraSet Brightness.vi"("Brightness"=9, "CameraDevRef"=w18) -> ("error out"=w15:errorcluster)  [unwired: 8 in, 1 out]
  n159 = while {
    tunnel: w68 -> [w296]
    tunnel: w67 -> [_]
    tunnel: [w299] -> _
    tunnel: w15 -> [_]
    tunnel: w4 -> [w286]
    tunnel: w3 -> [w285]
    i -> [w299]
    stop <- FALSE ("stop") stop-if-true
    n160 = disable-structure shown="Enabled" {
      disable-tunnel: [w300 "10.22.30.11" ("address")] -> w298
      frame Disabled {
        n161 = local read "Camera IP"() -> (w300:string)
      }
      frame Enabled {
      }
    }
    n162 = Select(t=enum16{"Read", "Reopen", "Close"}."Read" ("Operation"), s="Enable", f=enum16{"Read", "Reopen", "Close"}."Close" ("Operation")) -> (s? t:f=w292:enum16{"Read", "Reopen", "Close"})
    n163 = call <vilib>:"WPI_CameraRead MJPG.vi"("Operation"=w292, "Camera Settings"="Camera Settings", "Image"=w296, "address"=w298) -> ("error out"=w291:errorcluster, "Bandwidth (kbps)"=w294:dbl, "Image Out"=w295:T6)  [unwired: 5 in]
    n164 = Unbundle(w291) -> ("status"=w289:bool)  [unwired: 2 out]
    n165 = Compound Arithmetic op=AND("Enable", invert w289) -> (w288:bool)
    n166 = case shown="True" w288 {
      tunnel: "Camera Settings" -> [_ w324]
      tunnel: w295 -> [_ w327]
      tunnel: w294 -> [_ w326]
      tunnel: "Target Choice" -> [_ w311]
      tunnel: w286 -> [_ w308]
      tunnel: w285 -> [_ w316]
      frame False {
        # "Sleep for 500ms"
        n167 = Wait Until Next ms Multiple(millisecond multiple=u32 500) -> ()  [unwired: 1 out]
      }
      frame True {
        w317 = enum16{"206", "1011"}."1011"  # Camera Type
        # "Display image and save\nthe occasional frame to disk.\nThe image can also be processed here."
        # "Update Mbps\nindicator"
        n168 = case shown="4, 5" w326 {
          tunnel: [u32 6618880 ("Color Box") u32 16776722 ("Color Box") u32 16716800 ("Color Box")] -> w328
          frame Default {
          }
          frame 4, 5 {
          }
          frame 6.. {
          }
        }
        n169 = disable-structure shown="Enabled" {
          disable-tunnel: ["Color Plane" 1 ("Color Plane")] -> w318
          frame Enabled {
          }
          frame Disabled {
          }
        }
        n170 = Unbundle(w324) -> ("Frate Rate"=w323:i32)  [unwired: 2 out]
        n171 = call "FPS Calculator.vi"("Average Count"=w323) -> ("fps"=→"fps":dbl)  [unwired: 10 in]
        n172 = disable-structure shown="Enabled" {
          disable-tunnel: ["Range" cluster{"Lower value":sgl, "Upper value":sgl} {"Lower value"=120.0, "Upper value"=255.0} ("Range")] -> w314
          frame Enabled {
          }
          frame Disabled {
          }
        }
        n173 = Bundle("Color Box"=w328, "Color Box"=w328) -> (w330:cluster{"Color Box":u32, "Color Box":u32})  [unwired: 1 out]
        n174 = Build Array(w330) -> (w329:cluster{"Color Box":u32, "Color Box":u32}[])
        n175 = call "IMAQ Clear Overlay"("Image"=w327) -> ("error out"=w331:errorcluster, "Image Out"=w313:T6)  [unwired: 2 in, 7 out]
        n176 = property on="Mbps" class="Bool (strict)"("Colors [4]"=w329) -> ()  [unwired: 2 in, 2 out]
        n177 = Unbundle By Name(w331) -> ("status"=w332:bool)
        n178 = call "Target Analyze.vi"("Original Image_in"=w313, "Color Plane"=w318, "Range"=w314, "Camera Type"=w317, "Annotate"="Annotate", "Target Choice"=w311, "Mask"=w316, "gray"=w308) -> ("Numeric Target Info (X,Y,D)"=→"Position of Target's Center (x, y)":dbl[], "Target Info"=w309:T25, "Targert Found"=w310:bool, "Original Image_out+"=w312:T6, "Processed Image"=w306:T6, "Distance [m]"=w305:dbl, "Particle Scores"=w304:T26)  [unwired: 2 in, 3 out]
        "Camera Image" <- w312
        "Distance to Targets Center [m]" <- w305
        "Target Found" <- w310
        n179 = property on="Image Error Message" class="Str"("Visible"=w332) -> ()  [unwired: 2 in, 2 out]
        n180 = call "CCIP.vi"("Processed Image"=w306, "Distance (from camera to target)"=w305, "Particle Scores"=w304) -> ("Processed Image + aim markings"=→"Processed Image":T6)  [unwired: 12 in]
        n181 = call "Save DB Images.vi"("Image"=w312) -> ()  [unwired: 2 in, 1 out]
        n182 = call "Get Correct Target.vi"("2"="2", "3"="3", "Target Info"=w309, "Target Found?"=w310, "1"="1") -> ("Selected Target Info"=→"Selected Target Info":T8)  [unwired: 1 in]
        "Mbps" <- w326
      }
    }
  }
  n183 = call-poly <vilib>:"Read Key.vi"("section"=w43, "default value"=w44, "key"="Size", "refnum"=w46) -> ("value"=w33:string, "refnum out"=w28:T24)  [unwired: 2 in, 4 out]
  n184 = Read from Text File(file (use dialog)=w52, count=-1 ("timeout ms (25000)")) -> (refnum out=w30:refnum<file>, text=w53:string[], error out=w54:errorcluster)  [unwired: 2 in, 1 out]
  n185 = case shown="Error" w54 {
    tunnel: w53 -> [w341 _]
    tunnel: [w341 w343] -> w50
    tunnel: w51 -> [_ w343]
    tunnel: w52 -> [_ w344]
    tunnel: [w340 w342] -> w29
    tunnel: w30 -> [w340 _]
    frame No Error {
    }
    frame Error {
      n186 = Write to Text File(file (use dialog)=w344, text=w343) -> (refnum out=w342:refnum<file>)  [unwired: 2 in, 2 out]
    }
  }
  n187 = call-poly <vilib>:"Read Key.vi"("section"=w43, "default value"=30, "key"="FrameRate", "refnum"=w28) -> ("value"=w38:i32, "refnum out"=w27:T24)  [unwired: 1 in, 5 out]
  n188 = control-ref of="Tree"() -> (w24:refnum<vi>)
  n189 = property on="Listbox" class="LstBox (strict)"("Item Symbols"=i32[] [], "Item Names"=w50) -> ()  [unwired: 2 in, 2 out]
  n190 = Close File(refnum=w29) -> ()  [unwired: 1 in, 2 out]
  n191 = call-poly <vilib>:"Read Key.vi"("section"=w43, "default value"=30, "key"="Compression", "refnum"=w27) -> ("value"=w37:i32, "refnum out"=w25:T24)  [unwired: 1 in, 5 out]
  n192 = control-ref of="Test Tree"() -> (w23:refnum<vi>)
  n193 = while {
    tunnel: [w346] -> _
    tunnel: w24 -> [w345]
    i -> [w346]
    stop <- FALSE stop-if-true
    n194 = Wait (ms)(milliseconds to wait=u32 60) -> ()  [unwired: 1 out]
    n195 = case shown="\"Variables\"" "Viewer" {
      tunnel: w345 -> [_ w350]
      frame Default {
      }
      frame "Variables" {
        n196 = call <vilib>:"NT Read and Format Entries as Tree.vi"("Tree Refnum"=w350) -> ()  [unwired: 9 in, 2 out]
      }
    }
  }
  n197 = while {
    tunnel: w35 -> [w355]
    shift-right: [w354] -> _
    shift-left: w25 -> [w353]
    tunnel: [w352] -> _
    tunnel: w23 -> [w351]
    i -> [w352]
    stop <- FALSE stop-if-true
    n198 = event shown="[4] \"Listbox\": Double Click" {
      selector: _ -> [_ _ _ _ _ _ _ _ _ _ _ _ _]
      dyn-events: _ -> [_ _ _ _ _ _ _ _ _ _ _ _ _]
      timeout: u32 60 ("milliseconds to wait") -> [_ _ _ _ _ _ _ _ _ _ _ _ _]
      tunnel: w351 -> [w365 _ _ _ _ _ _ _ _ _ _ _ _]
      tunnel: "Test Tree" -> [_ _ _ _ _ _ _ _ w559 w567 w569 w573 w581]
      tunnel: w355 -> [_ w387 _ _ _ _ w523 w553 _ _ _ _ _]
      tunnel: [w359 w386 _ w489 w497 w509 w522 w546 w558 w565 w568 w572 w580] -> w354
      tunnel: w353 -> [w359 w386 _ w489 w497 w509 w521 w546 w558 w565 w568 w572 w580]
      event Timeout {
        w364 = enum16{"Update", "Clear"}[] [enum."Clear", enum."Clear", enum."Clear", enum."Clear", enum."Update", enum."Update", enum."Clear"] items=["Update", "Clear"]
        n199 = event-data() -> ()  [unwired: 1 in, 1 out]
        n200 = local read "Mode"() -> (w362:T2)
        n201 = Index Array(array=w364, index=w362) -> (element=w363:enum16{"Update", "Clear"})
        n202 = call <vilib>:"NT Read String.vi"("Name"="TestMode/TestName") -> ("String"=w368:string)  [unwired: 9 in, 1 out]
        n203 = case shown="\"Operation\", Default" "Dashboard Tab" {
          tunnel: w365 -> [_ w378]
          tunnel: "/TestMode/Automatic/" ("Name Pattern") -> [_ w377]
          tunnel: w363 -> [_ w376]
          tunnel: w362 -> [_ w374]
          frame "Operation", Default {
          }
          frame "Test" {
            w373 = -2 ("Active Item:Row Number")
            n204 = call <vilib>:"NT Read and Format Entries as Tree.vi"("Operation"=w376, "Name Pattern"=w377, "Tree Refnum"=w378) -> ()  [unwired: 7 in, 2 out]
            n205 = Index Array(array=u32[] [14013909, 14013909, 14013909, 14013909, 14013909, 16777215, 14013909], index=w374) -> (element=w372:u32)
            n206 = property on="Test Tree" class="Tree (strict)"("Active Item Row Number"=w373, "ActiveColNum"=w373, "CellBG"=w372, "Active Item Row Number"=-1 ("Active Item:Row Number"), "CellBG"=u32 5789784 ("Color Box")) -> ()  [unwired: 2 in, 2 out]
          }
        }
        n207 = case shown="\"\"" w368 {
          tunnel: "TestMode/TestProgress" ("Name") -> [w380 _]
          tunnel: "TestMode/TestProgressText" ("Name") -> [w379 _]
          frame Default {
            n208 = call <vilib>:"NT Read Number.vi"("Name"=w380) -> ("Numeric"=w381:dbl)  [unwired: 9 in, 1 out]
            n209 = call <vilib>:"NT Read String.vi"("Name"=w379) -> ("String"=w382:string)  [unwired: 9 in, 1 out]
            n210 = Bundle("Numeric"=w381, "String"=w382) -> (→"Progress":cluster{"Numeric":dbl, "String":string})  [unwired: 1 in]
          }
          frame "" {
            n211 = property on="Progress" class="Clust (strict)"("Visible"=FALSE) -> ()  [unwired: 2 in, 2 out]
            n212 = local write "Test Name"(u16 0) -> ()
          }
        }
      }
      event "Test Tree": Value Change {
        # "Show appropriate\ncontrols"
        n213 = event-data() -> ("CtlRef"=w390:refnum<vi>, "NewVal"=w388:string)  [unwired: 1 in]
        n214 = call <vilib>:"WPI_UtilitiesGetTreeIOName.vi"("NewVal"=w388, "TreeControl in"=w390) -> ("I/O Name"=w391:string)  [unwired: 9 in]
        n215 = case shown="\"Camera\"" w391 {
          selector: w391 -> [_ w398 _ w416 w425 _]
          tunnel: w388 -> [_ _ w413 w415 _ w432]
          tunnel: w387 -> [_ _ _ _ _ w431]
          frame Default {
            w393 = FALSE ("Visible")
            w392 = FALSE ("Visible")
            n216 = property on="Motor" class="Clust (strict)"("Visible"=w392) -> ()  [unwired: 2 in, 2 out]
            n217 = property on="Ring" class="Ring (strict)"("Visible"=w392) -> ()  [unwired: 2 in, 2 out]
            n218 = property on="Rev/Fwd" class="Clust (strict)"("Visible"=w393) -> ()  [unwired: 2 in, 2 out]
            n219 = property on="On/Off" class="Bool (strict)"("Visible"=w393) -> ()  [unwired: 2 in, 2 out]
            n220 = property on="Slider" class="Slide (strict)"("Visible"=w393) -> ()  [unwired: 2 in, 2 out]
          }
          frame "Motor", "PWM" {
            w399 = FALSE ("Visible")
            n221 = case shown="\"Motor\", Default" w398 {
              tunnel: [1.0 ("Value") -1.0 ("Value")] -> w397
              tunnel: [255.0 ("Value") 1.0 ("Value")] -> w396
              tunnel: [128.0 ("Value") 0.0 ("Value")] -> w395
              tunnel: [64.0 ("Value") 0.5 ("Value")] -> w394
              frame "PWM" {
              }
              frame "Motor", Default {
              }
            }
            n222 = property on="Motor" class="Clust (strict)"("Visible"=TRUE) -> ()  [unwired: 2 in, 2 out]
            n223 = property on="Value" class="Slide (strict)"("Value"=w395, "Scale.Minimum"=w397, "Scale.Maximum"=w396, "Scale.Increment"=w394) -> ()  [unwired: 2 in, 2 out]
            n224 = property on="On/Off" class="Bool (strict)"("Visible"=w399) -> ()  [unwired: 2 in, 2 out]
            n225 = property on="Slider" class="Slide (strict)"("Visible"=w399) -> ()  [unwired: 2 in, 2 out]
            n226 = property on="Ring" class="Ring (strict)"("Visible"=w399) -> ()  [unwired: 2 in, 2 out]
            n227 = property on="Rev/Fwd" class="Clust (strict)"("Visible"=w399) -> ()  [unwired: 2 in, 2 out]
          }
          frame "Servo" {
            w411 = FALSE ("Visible")
            n228 = call <vilib>:"NT Read Number.vi"("Name"=w413) -> ("Numeric"=w412:dbl)  [unwired: 9 in, 1 out]
            n229 = property on="Slider" class="Slide (strict)"("Visible"=TRUE, "Scale.Maximum"=170.0 ("Scale.Range:Maximum")) -> ()  [unwired: 2 in, 2 out]
            n230 = local write "Slider"(w412) -> ()
            n231 = property on="Motor" class="Clust (strict)"("Visible"=w411) -> ()  [unwired: 2 in, 2 out]
            n232 = property on="Rev/Fwd" class="Clust (strict)"("Visible"=w411) -> ()  [unwired: 2 in, 2 out]
            n233 = property on="On/Off" class="Bool (strict)"("Visible"=w411) -> ()  [unwired: 2 in, 2 out]
            n234 = property on="Ring" class="Ring (strict)"("Visible"=w411) -> ()  [unwired: 2 in, 2 out]
          }
          frame "Relay", "Solenoid" {
            w414 = FALSE ("Visible")
            n235 = property on="Motor" class="Clust (strict)"("Visible"=w414) -> ()  [unwired: 2 in, 2 out]
            n236 = property on="Slider" class="Slide (strict)"("Visible"=w414) -> ()  [unwired: 2 in, 2 out]
            n237 = Search and Replace String(input string=w415, search string="/Value  **", replace string="/Direction") -> (result string=w421:string)  [unwired: 5 in, 3 out]
            n238 = property on="Ring" class="Ring (strict)"("Visible"=w414) -> ()  [unwired: 2 in, 2 out]
            n239 = call <vilib>:"NT Read String.vi"("Name"=w421) -> ("String"=w419:string)  [unwired: 9 in, 1 out]
            n240 = Equal?(x="Both directions", y=w419) -> (x = y?=w417:bool)
            n241 = Not(x=w417) -> (.not. x?=w418:bool)
            n242 = property on="Rev/Fwd" class="Clust (strict)"("Visible"=w417) -> ()  [unwired: 2 in, 2 out]
            n243 = property on="On/Off" class="Bool (strict)"("Visible"=w418, "Caption.Text"=w416) -> ()  [unwired: 2 in, 2 out]
          }
          frame "Compressor", "Digital Out" {
            w424 = FALSE ("Visible")
            # "Get direction and finish"
            n244 = property on="Motor" class="Clust (strict)"("Visible"=w424) -> ()  [unwired: 2 in, 2 out]
            n245 = property on="Slider" class="Slide (strict)"("Visible"=w424) -> ()  [unwired: 2 in, 2 out]
            n246 = property on="Ring" class="Ring (strict)"("Visible"=w424) -> ()  [unwired: 2 in, 2 out]
            n247 = property on="On/Off" class="Bool (strict)"("Visible"=TRUE, "Caption.Text"=w425) -> ()  [unwired: 2 in, 2 out]
            n248 = property on="Rev/Fwd" class="Clust (strict)"("Visible"=FALSE) -> ()  [unwired: 2 in, 2 out]
          }
          frame "Camera" {
            n249 = call <vilib>:"Get Last Path Segment.vi"("String in"=w432) -> ("String out"=w433:string)  [unwired: 10 in]
            n250 = property on="On/Off" class="Bool (strict)"("Visible"=FALSE) -> ()  [unwired: 2 in, 2 out]
            n251 = property on="Motor" class="Clust (strict)"("Visible"=FALSE) -> ()  [unwired: 2 in, 2 out]
            n252 = property on="Rev/Fwd" class="Clust (strict)"("Visible"=FALSE) -> ()  [unwired: 2 in, 2 out]
            n253 = case shown="\"White Balance  **\"" w433 {
              tunnel: w432 -> [w439 w448 w457 w466 w475 _ w481]
              tunnel: w431 -> [w437 w445 w454 w463 w472 _ _]
              frame "Size  **" {
                n254 = Index Array(array=w437) -> (element=w436:cluster{string[]})  [unwired: 1 in]
                n255 = call <vilib>:"NT Read String.vi"("Name"=w439) -> ("String"=w438:string)  [unwired: 9 in, 1 out]
                n256 = Unbundle(w436) -> (w434:string[])
                n257 = Match First String(2:w434, 3:w438) -> (0:w435:i32)  [unwired: 1 out]
                n258 = property on="Ring" class="Ring (strict)"("Value"=w435, "Strings []"=w434) -> ()  [unwired: 2 in, 2 out]
                n259 = property on="Ring" class="Ring (strict)"("Visible"=TRUE) -> ()  [unwired: 2 in, 2 out]
                n260 = property on="Slider" class="Slide (strict)"("Visible"=FALSE) -> ()  [unwired: 2 in, 2 out]
              }
              frame "White Balance  **" {
                n261 = Index Array(array=w445, index=1) -> (element=w446:cluster{string[]})
                n262 = call <vilib>:"NT Read String.vi"("Name"=w448) -> ("String"=w447:string)  [unwired: 9 in, 1 out]
                n263 = Unbundle(w446) -> (w443:string[])
                n264 = Match First String(2:w443, 3:w447) -> (0:w442:i32)  [unwired: 1 out]
                n265 = property on="Ring" class="Ring (strict)"("Value"=w442, "Strings []"=w443) -> ()  [unwired: 2 in, 2 out]
                n266 = property on="Ring" class="Ring (strict)"("Visible"=TRUE) -> ()  [unwired: 2 in, 2 out]
                n267 = property on="Slider" class="Slide (strict)"("Visible"=FALSE) -> ()  [unwired: 2 in, 2 out]
              }
              frame "Exposure  **" {
                n268 = Index Array(array=w454, index=2) -> (element=w455:cluster{string[]})
                n269 = call <vilib>:"NT Read String.vi"("Name"=w457) -> ("String"=w456:string)  [unwired: 9 in, 1 out]
                n270 = Unbundle(w455) -> (w451:string[])
                n271 = Match First String(2:w451, 3:w456) -> (0:w452:i32)  [unwired: 1 out]
                n272 = property on="Ring" class="Ring (strict)"("Value"=w452, "Strings []"=w451) -> ()  [unwired: 2 in, 2 out]
                n273 = property on="Ring" class="Ring (strict)"("Visible"=TRUE) -> ()  [unwired: 2 in, 2 out]
                n274 = property on="Slider" class="Slide (strict)"("Visible"=FALSE) -> ()  [unwired: 2 in, 2 out]
              }
              frame "Exposure Priority  **" {
                n275 = Index Array(array=w463, index=3) -> (element=w464:cluster{string[]})
                n276 = call <vilib>:"NT Read String.vi"("Name"=w466) -> ("String"=w465:string)  [unwired: 9 in, 1 out]
                n277 = Unbundle(w464) -> (w460:string[])
                n278 = Match First String(2:w460, 3:w465) -> (0:w461:i32)  [unwired: 1 out]
                n279 = property on="Ring" class="Ring (strict)"("Value"=w461, "Strings []"=w460) -> ()  [unwired: 2 in, 2 out]
                n280 = property on="Ring" class="Ring (strict)"("Visible"=TRUE) -> ()  [unwired: 2 in, 2 out]
                n281 = property on="Slider" class="Slide (strict)"("Visible"=FALSE) -> ()  [unwired: 2 in, 2 out]
              }
              frame "Color Enable  **" {
                n282 = Index Array(array=w472, index=4) -> (element=w473:cluster{string[]})
                n283 = call <vilib>:"NT Read String.vi"("Name"=w475) -> ("String"=w474:string)  [unwired: 9 in, 1 out]
                n284 = Unbundle(w473) -> (w469:string[])
                n285 = Match First String(2:w469, 3:w474) -> (0:w470:i32)  [unwired: 1 out]
                n286 = property on="Ring" class="Ring (strict)"("Value"=w470, "Strings []"=w469) -> ()  [unwired: 2 in, 2 out]
                n287 = property on="Ring" class="Ring (strict)"("Visible"=TRUE) -> ()  [unwired: 2 in, 2 out]
                n288 = property on="Slider" class="Slide (strict)"("Visible"=FALSE) -> ()  [unwired: 2 in, 2 out]
              }
              frame Default {
                n289 = property on="Ring" class="Ring (strict)"("Visible"=FALSE) -> ()  [unwired: 2 in, 2 out]
                n290 = property on="Slider" class="Slide (strict)"("Visible"=FALSE) -> ()  [unwired: 2 in, 2 out]
              }
              frame "Brightness  **", "Color Level  **", "Compression  **", "FPS  **", "Sharpness  **" {
                n291 = call <vilib>:"NT Read Number.vi"("Name"=w481) -> ("Numeric"=w480:dbl)  [unwired: 9 in, 1 out]
                n292 = local write "Slider"(w480) -> ()
                n293 = property on="Slider" class="Slide (strict)"("Visible"=TRUE, "Scale.Maximum"=100.0 ("Scale.Range:Maximum")) -> ()  [unwired: 2 in, 2 out]
                n294 = property on="Ring" class="Ring (strict)"("Visible"=FALSE) -> ()  [unwired: 2 in, 2 out]
              }
            }
          }
        }
        n295 = property on="Progress" class="Clust (strict)"("Visible"=FALSE) -> ()  [unwired: 2 in, 2 out]
      }
      event "Test Name": Mouse Enter {
        # "Populate the ring with the list of tests"
        n296 = event-data() -> ()  [unwired: 1 in, 1 out]
        n297 = call <vilib>:"NT Read String Array.vi"("Name"="TestMode/TestList") -> ("String Array"=w488:string[])  [unwired: 9 in, 1 out]
        n298 = Build Array (concatenate)("Select the test to run...", w488) -> (w487:string[])
        n299 = property on="Test Name" class="Ring (strict)"("Strings []"=w487) -> ()  [unwired: 2 in, 2 out]
      }
      event "Test Name": Value Change {
        w490 = FALSE ("Visible")
        # "Tell the robot the test name to run"
        n300 = event-data() -> ("NewVal"=w494:u16)  [unwired: 1 in]
        n301 = property on="Test Name" class="Ring (strict)"() -> ("Strings []"=w495:string[])  [unwired: 2 in, 2 out]
        n302 = local write "Progress"(T7 {"Test Progress"=0, "Test Progress Text"=""} ("Progress")) -> ()
        n303 = Index Array(array=w495, index=w494) -> (element=w493:string)
        n304 = call <vilib>:"NT Write String.vi"("String"=w493, "Name"="TestMode/TestName") -> ()  [unwired: 9 in, 1 out]
        n305 = property on="Progress" class="Clust (strict)"("Visible"=TRUE) -> ()  [unwired: 2 in, 2 out]
        n306 = property on="Motor" class="Clust (strict)"("Visible"=w490) -> ()  [unwired: 2 in, 2 out]
        n307 = property on="Slider" class="Slide (strict)"("Visible"=w490) -> ()  [unwired: 2 in, 2 out]
        n308 = property on="On/Off" class="Bool (strict)"("Visible"=w490) -> ()  [unwired: 2 in, 2 out]
        n309 = property on="Rev/Fwd" class="Clust (strict)"("Visible"=w490) -> ()  [unwired: 2 in, 2 out]
        n310 = property on="Ring" class="Ring (strict)"("Visible"=w490) -> ()  [unwired: 2 in, 2 out]
      }
      event "Listbox": Double Click {
        n311 = event-data() -> ("PlatMods.Shift"=w498:bool, "Row"=w500:i32)  [unwired: 1 in]
        n312 = case shown="False" w498 {
          tunnel: w500 -> [w504 _]
          tunnel: 1 -> [w503 _]
          frame False {
            n313 = property on="Listbox" class="LstBox (strict)"() -> ("Item Symbols"=w502:i32[])  [unwired: 2 in, 2 out]
            n314 = Replace Array Subset(array=w502, new element=w503, index=w504) -> (w501:i32[])
            n315 = property on="Listbox" class="LstBox (strict)"("Item Symbols"=w501) -> ()  [unwired: 2 in, 2 out]
          }
          frame True {
            w505 = 0 ("Top Row")
            n316 = property on="Listbox" class="LstBox (strict)"() -> ("Number of Rows"=w507:u32)  [unwired: 2 in, 2 out]
            n317 = Initialize Array(0, w507) -> (w506:i32[])
            n318 = property on="Listbox" class="LstBox (strict)"("Top Row"=w505, "Value"=w505, "Item Symbols"=w506) -> ()  [unwired: 2 in, 2 out]
          }
        }
      }
      event "Listbox": Key Down {
        n319 = event-data() -> ("VKey"=w511:T27)  [unwired: 1 in]
        n320 = case shown="\"Left\", \"Right\"" w511 {
          selector: w511 -> [w516 _]
          tunnel: eventvkey."Left" ("VKey") -> [w514 _]
          frame "Left", "Right" {
            n321 = Equal?(x=w514, y=w516) -> (x = y?=w515:bool)
            n322 = Select(t=0, s=w515, f=1) -> (s? t:f=w517:i32)
            n323 = property on="Listbox" class="LstBox (strict)"() -> ("Item Symbols"=w520:i32[])  [unwired: 2 in, 2 out]
            n324 = Replace Array Subset(array=w520, new element=w517, index="Listbox") -> (w519:i32[])
            n325 = property on="Listbox" class="LstBox (strict)"("Item Symbols"=w519) -> ()  [unwired: 2 in, 2 out]
          }
          frame Default {
          }
        }
      }
      event "DB Camera Config": Value Change {
        n326 = event-data() -> ("NewVal"=w524:bool)  [unwired: 1 in]
        n327 = case shown="False" w524 {
          tunnel: w523 -> [w533 _]
          tunnel: [w526 w544] -> w522
          tunnel: w521 -> [w525 w544]
          frame False {
            w540 = "Camera"
            w543 = FALSE ("Visible")
            n328 = local read "Camera Settings"() -> (w532:T1)
            n329 = Index Array(array=w533) -> (element=w536:cluster{string[]})  [unwired: 1 in]
            n330 = Unbundle(w532) -> ("Frate Rate"=w531:i32, "Compression"=w530:i32, "Size"=w534:u16)
            n331 = Unbundle(w536) -> (w535:string[])
            n332 = Index Array(array=w535, index=w534) -> (element=w529:string)
            n333 = call-poly <vilib>:"Write Key.vi"("section"=w540, "value"=w529, "key"="Size", "refnum"=w525) -> ("refnum out"=w542:T24)  [unwired: 2 in, 5 out]
            n334 = call-poly <vilib>:"Write Key.vi"("section"=w540, "value"=w531, "key"="FrameRate", "refnum"=w542) -> ("refnum out"=w541:T24)  [unwired: 1 in, 6 out]
            n335 = property on="Camera Settings" class="Clust (strict)"("Visible"=w543) -> ()  [unwired: 2 in, 2 out]
            n336 = local write "DB Camera Config"(w543) -> ()
            n337 = call-poly <vilib>:"Write Key.vi"("section"=w540, "value"=w530, "key"="Compression", "refnum"=w541) -> ("refnum out"=w527:T24)  [unwired: 1 in, 6 out]
            n338 = call <vilib>:"Close Config Data.vi"("refnum"=w527) -> ("file path"=w528:path)  [unwired: 2 in, 8 out]
            n339 = call <vilib>:"Open Config Data.vi"("configuration file path"=w528) -> ("refnum"=w526:T24)  [unwired: 8 in, 2 out]
          }
          frame True {
            n340 = property on="Camera Settings" class="Clust (strict)"("Visible"=TRUE) -> ()  [unwired: 2 in, 2 out]
          }
        }
      }
      event "Camera Settings": Value Change {
        n341 = event-data() -> ("NewVal"=w557:T1)  [unwired: 1 in]
        n342 = Index Array(array=w553) -> (element=w552:cluster{string[]})  [unwired: 1 in]
        n343 = Unbundle(w557) -> ("Frate Rate"=w548:i32, "Compression"=w547:i32, "Size"=w550:u16)
        n344 = Unbundle(w552) -> (w551:string[])
        n345 = Index Array(array=w551, index=w550) -> (element=w549:string)
        n346 = Format Into String(format string="%s   %dfps   %d%%", w549, w548, w547) -> (resulting string=w554:string)  [unwired: 2 in, 1 out]
        n347 = Build Array(w554) -> (w555:string[])
        n348 = property on="DB Camera Config" class="Bool (strict)"("Strings [4]"=w555) -> ()  [unwired: 2 in, 2 out]
      }
      event "Motor.Enable": Value Change {
        n349 = event-data() -> ("NewVal"=w563:bool)  [unwired: 1 in]
        n350 = Unbundle("Motor") -> ("Value"=w562:dbl)  [unwired: 1 out]
        n351 = Select(t=w562, s=w563, f=0.0) -> (s? t:f=w560:dbl)
        n352 = call <vilib>:"NT Write Number.vi"("Numeric"=w560, "Name"=w559) -> ()  [unwired: 9 in, 1 out]
      }
      event "Slider": Value Change {
        n353 = event-data() -> ("NewVal"=w566:dbl)  [unwired: 1 in]
        n354 = call <vilib>:"NT Write Number.vi"("Numeric"=w566, "Name"=w567) -> ()  [unwired: 9 in, 1 out]
      }
      event "On/Off": Value Change {
        n355 = event-data() -> ("NewVal"=w571:bool)  [unwired: 1 in]
        n356 = Boolean To (0,1)(Boolean=w571) -> (0, 1=w570:i16)
        n357 = call <vilib>:"NT Write Number.vi"("Numeric"=w570, "Name"=w569) -> ()  [unwired: 9 in, 1 out]
      }
      event "Rev/Fwd": Value Change {
        n358 = event-data() -> ("NewVal.Forward"=w579:bool, "NewVal.Reverse"=w578:bool)  [unwired: 1 in]
        n359 = Boolean To (0,1)(Boolean=w579) -> (0, 1=w575:i16)
        n360 = Boolean To (0,1)(Boolean=w578) -> (0, 1=w577:i16)
        n361 = Negate(x=w577) -> (-x=w576:i16)
        n362 = Add(x=w575, y=w576) -> (x+y=w574:i16)
        n363 = call <vilib>:"NT Write Number.vi"("Numeric"=w574, "Name"=w573) -> ()  [unwired: 9 in, 1 out]
      }
      event "Ring": Value Change {
        n364 = event-data() -> ("NewVal"=w583:u16)  [unwired: 1 in]
        n365 = property on="Ring" class="Ring (strict)"() -> ("Strings []"=w584:string[])  [unwired: 2 in, 2 out]
        n366 = Index Array(array=w584, index=w583) -> (element=w582:string)
        n367 = call <vilib>:"NT Write String.vi"("String"=w582, "Name"=w581) -> ()  [unwired: 9 in, 1 out]
      }
    }
  }
  n368 = Index Array(array=w35) -> (element=w36:cluster{string[]})  [unwired: 1 in]
  n369 = property on="On/Off" class="Bool (strict)"("Visible"=w49) -> ()  [unwired: 2 in, 2 out]
  n370 = property on="Motor" class="Clust (strict)"("Visible"=w49) -> ()  [unwired: 2 in, 2 out]
  n371 = property on="Progress" class="Clust (strict)"("Visible"=w49) -> ()  [unwired: 2 in, 2 out]
  n372 = property on="Ring" class="Ring (strict)"("Visible"=w49) -> ()  [unwired: 2 in, 2 out]
  n373 = property on="Rev/Fwd" class="Clust (strict)"("Visible"=w49) -> ()  [unwired: 2 in, 2 out]
  n374 = Unbundle(w36) -> (w34:string[])
  n375 = Match First String(2:w34, 3:w33) -> (0:w32:i32)  [unwired: 1 out]
  n376 = Bundle("value"=w38, "value"=w37, "index"=w32) -> (w26:cluster{"value":i32, "value":i32, "index":i32})  [unwired: 1 out]
  n377 = property on="Camera Settings" class="Clust (strict)"("Val(Sgnl)"=w26) -> ()  [unwired: 2 in, 2 out]
  n378 = property on="Camera Settings" class="Clust (strict)"("Visible"=w49) -> ()  [unwired: 2 in, 2 out]
  n379 = local write "DB Camera Config"(w49) -> ()
  n380 = disable-structure shown="Enabled" {
    frame Disabled {
      # "Terminals of controls and indicators\nthat are bound to the smart dashboard by name.\nYou can place them anywhere you like and\neven read data from them."
    }
    frame Enabled {
    }
  }
